vi "Pause I2C Messages.vi"(8 "error in (no error)":errorcluster, 11 "PauseResume Ref":refnum<vi>) -> (0 "error out":errorcluster, 2 "I2C Messages":string[][](array[string]))   [LabVIEW 2025, in "I2C Bus Monitor UI.lvlib"]
uses:
  I2C Bus Monitor UI.lvlib
  Table Buffer - Dequeue.vi
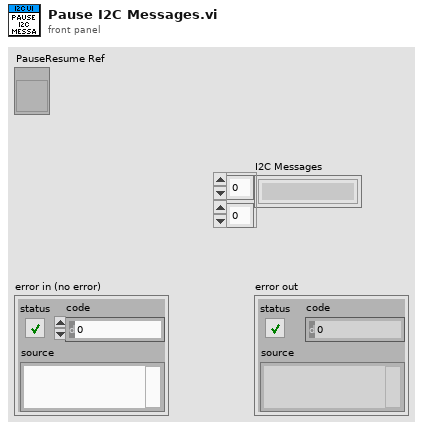
[diagram p1: front panel]
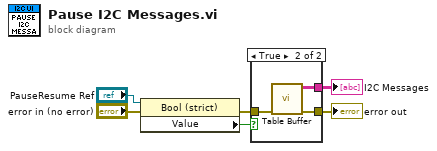
[diagram p0: block diagram]
diagram:
  n1 = property class="Bool (strict)"(reference="PauseResume Ref", error in="error in (no error)") -> (error out=w4:errorcluster, "Value"=w2:bool)  [unwired: 1 out]
  n2 = case shown="True" w2 {
    tunnel: [w7 w10] -> w6
    tunnel: w4 -> [w7 w9]
    tunnel: [_ w8] -> w1
    frame False {
    }
    frame True {
      n3 = call-poly "Table Buffer.vi"("error in (no error)"=w9) -> ("error out"=w10:errorcluster, "Data"=w8:string[][])  [unwired: 9 in]
    }
  }
  "error out" <- w6
  "I2C Messages" <- w1
